vi "MessageQueue_DequeueElement.vi"(0 "QueueIn":refnum<queue>, 2 "Timeout":i32=-1, 5 "ErrorIn":errorcluster) -> (14 "QueueOut":refnum<queue>, 16 "Message":string, 17 "Data":variant, 18 "Timeout":bool, 19 "ErrorOut":errorcluster)   [LabVIEW 2016]
doc: "Holt sich ein Element aus der Queue\n\nsige / 4.12.13"
uses:
  private/MessageQueue.MessageTypeDef.ctl
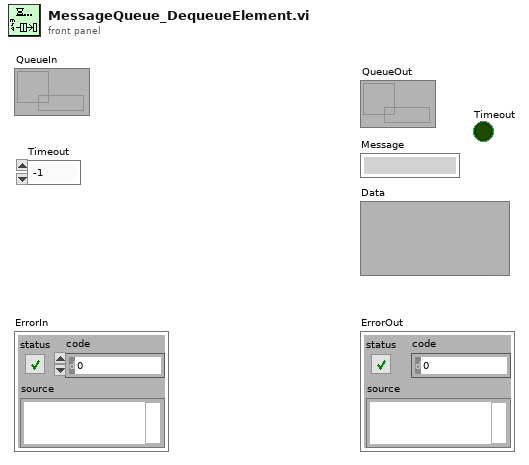
[diagram p1: front panel]
types:
  T1 = typedef "MessageQueue.MessageTypeDef.ctl" = cluster{"Message":string, "Data":variant}
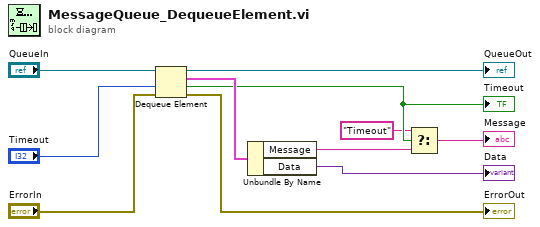
[diagram p0: block diagram]
diagram:
  n1 = Dequeue Element(queue="QueueIn", timeout in ms (-1)="Timeout", error in (no error)="ErrorIn") -> (queue out=→"QueueOut":refnum<queue>, element=w7:T1, timed out?=w4:bool, error out=→"ErrorOut":errorcluster)
  "Timeout" <- w4
  n2 = Unbundle By Name(w7) -> ("Message"=w3:string, "Data"=→"Data":variant)
  n3 = Select(t="Timeout", s=w4, f=w3) -> (s? t:f=→"Message":string)
